vi "decodeStream.vi"(8 "error in (no error)":errorcluster, 9 "beginIndex":i32, 10 "binary stream":u8[](array[numeric]), 11 "tBSON_I64 in":refnum<class "tBSON_I64.lvclass">) -> (0 "error out":errorcluster, 1 "endIndex":i32, 2 "binary stream out":u8[](array[numeric]), 3 "tBSON_I64 out":refnum<class "tBSON_I64.lvclass">)   [LabVIEW 2013, in "BSON.lvlib" / "tBSON_I64.lvclass"]
uses:
  tBSON_I64.lvclass
  tBSONElement/tBSONElement.lvclass
  setValue.vi
  BSON.lvlib
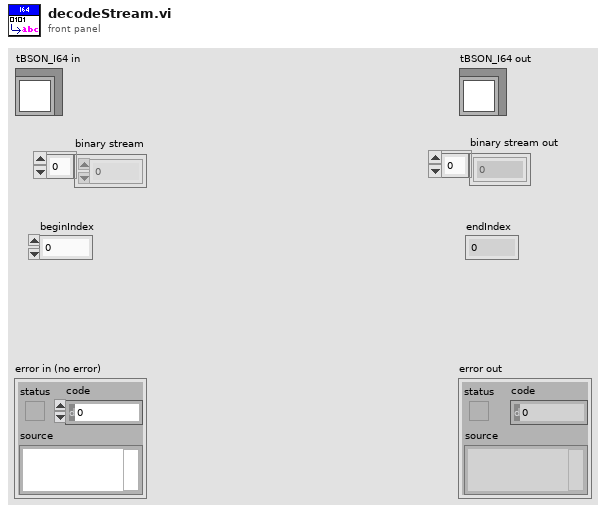
[diagram p1: front panel]
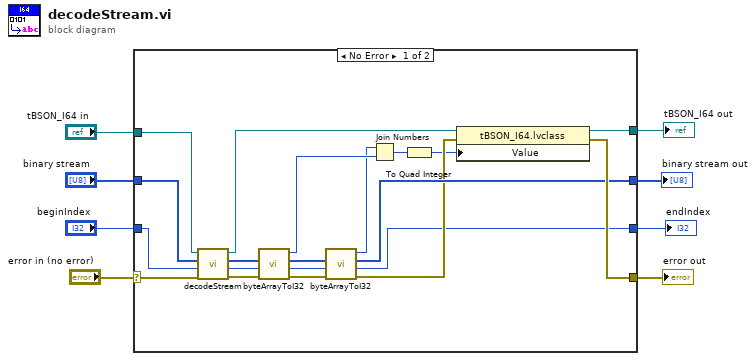
[diagram p0: block diagram]
diagram:
  n1 = case shown="No Error" "error in (no error)" {
    selector: "error in (no error)" -> [w28 w32]
    tunnel: [w23 w32] -> w4
    tunnel: "beginIndex" -> [w26 w31]
    tunnel: [w11 w31] -> w3
    tunnel: "binary stream" -> [w25 w30]
    tunnel: [w15 w30] -> w2
    tunnel: "tBSON_I64 in" -> [w27 w29]
    tunnel: [w22 w29] -> w1
    frame No Error {
      n2 = call-parent "decodeStream.vi"("error in (no error)"=w28, "beginIndex"=w26, "binary stream"=w25, "tBSONElement in"=w27) -> ("error out"=w21:errorcluster, "endIndex"=w19:i32, "binary stream out"=w20:u8[], "tBSONElement out"=w24:refnum<class "tBSON_I64.lvclass">)  [unwired: 4 in]
      n3 = call "byteArrayToI32.vi"("error in (no error)"=w21, "StartIndex"=w19, "ByteArrayIn"=w20) -> ("error out"=w16:errorcluster, "EndIndex"=w17:i32, "ByteArrayOut"=w18:u8[], "I32"=w14:i32)  [unwired: 5 in]
      n4 = call "byteArrayToI32.vi"("error in (no error)"=w16, "StartIndex"=w17, "ByteArrayIn"=w18) -> ("error out"=w12:errorcluster, "EndIndex"=w11:i32, "ByteArrayOut"=w15:u8[], "I32"=w13:i32)  [unwired: 5 in]
      n5 = Join Numbers(hi=w13, lo=w14) -> ((hi.lo)=w10:u64)
      n6 = To Quad Integer(1:w10) -> (0:w9:i64)
      n7 = property class="tBSON_I64.lvclass"(reference=w24, error in=w12, "Value"=w9) -> (reference out=w22:refnum<class "tBSON_I64.lvclass">, error out=w23:errorcluster)
    }
    frame Error {
    }
  }
  "error out" <- w4
  "tBSON_I64 out" <- w1
  "binary stream out" <- w2
  "endIndex" <- w3
